vi "xcorr bkp.vi"(4 "shift":u8, 6 "N":u8, 7 "y":u32, 8 "x":u32, 9 "enable":bool, 10 "lag":u16) -> (1 "Rxy valid":bool, 2 "Rxy":u64, 3 "trigger":bool)   [LabVIEW 2017]
uses:
  <vilib>/rvi/FXPMathLib/basic elements/FxpDiscreteDelay/XNode/nifxpmath_DiscreteDelay.xnode
panel:
  in  "Pulse Energy":fxp<+,48,0>=0.99609375
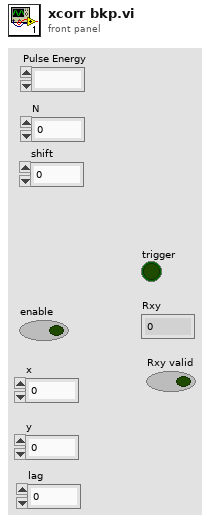
[diagram p1: front panel]
types:
  T1 = cluster{"Q":bool, "Q":bool, "Q":bool, "Q":bool, "Q":bool, "Q":bool, "Q":bool, "Q":bool, "Q":bool, "Q":bool, "Q":bool, "Q":bool, "valid":bool}
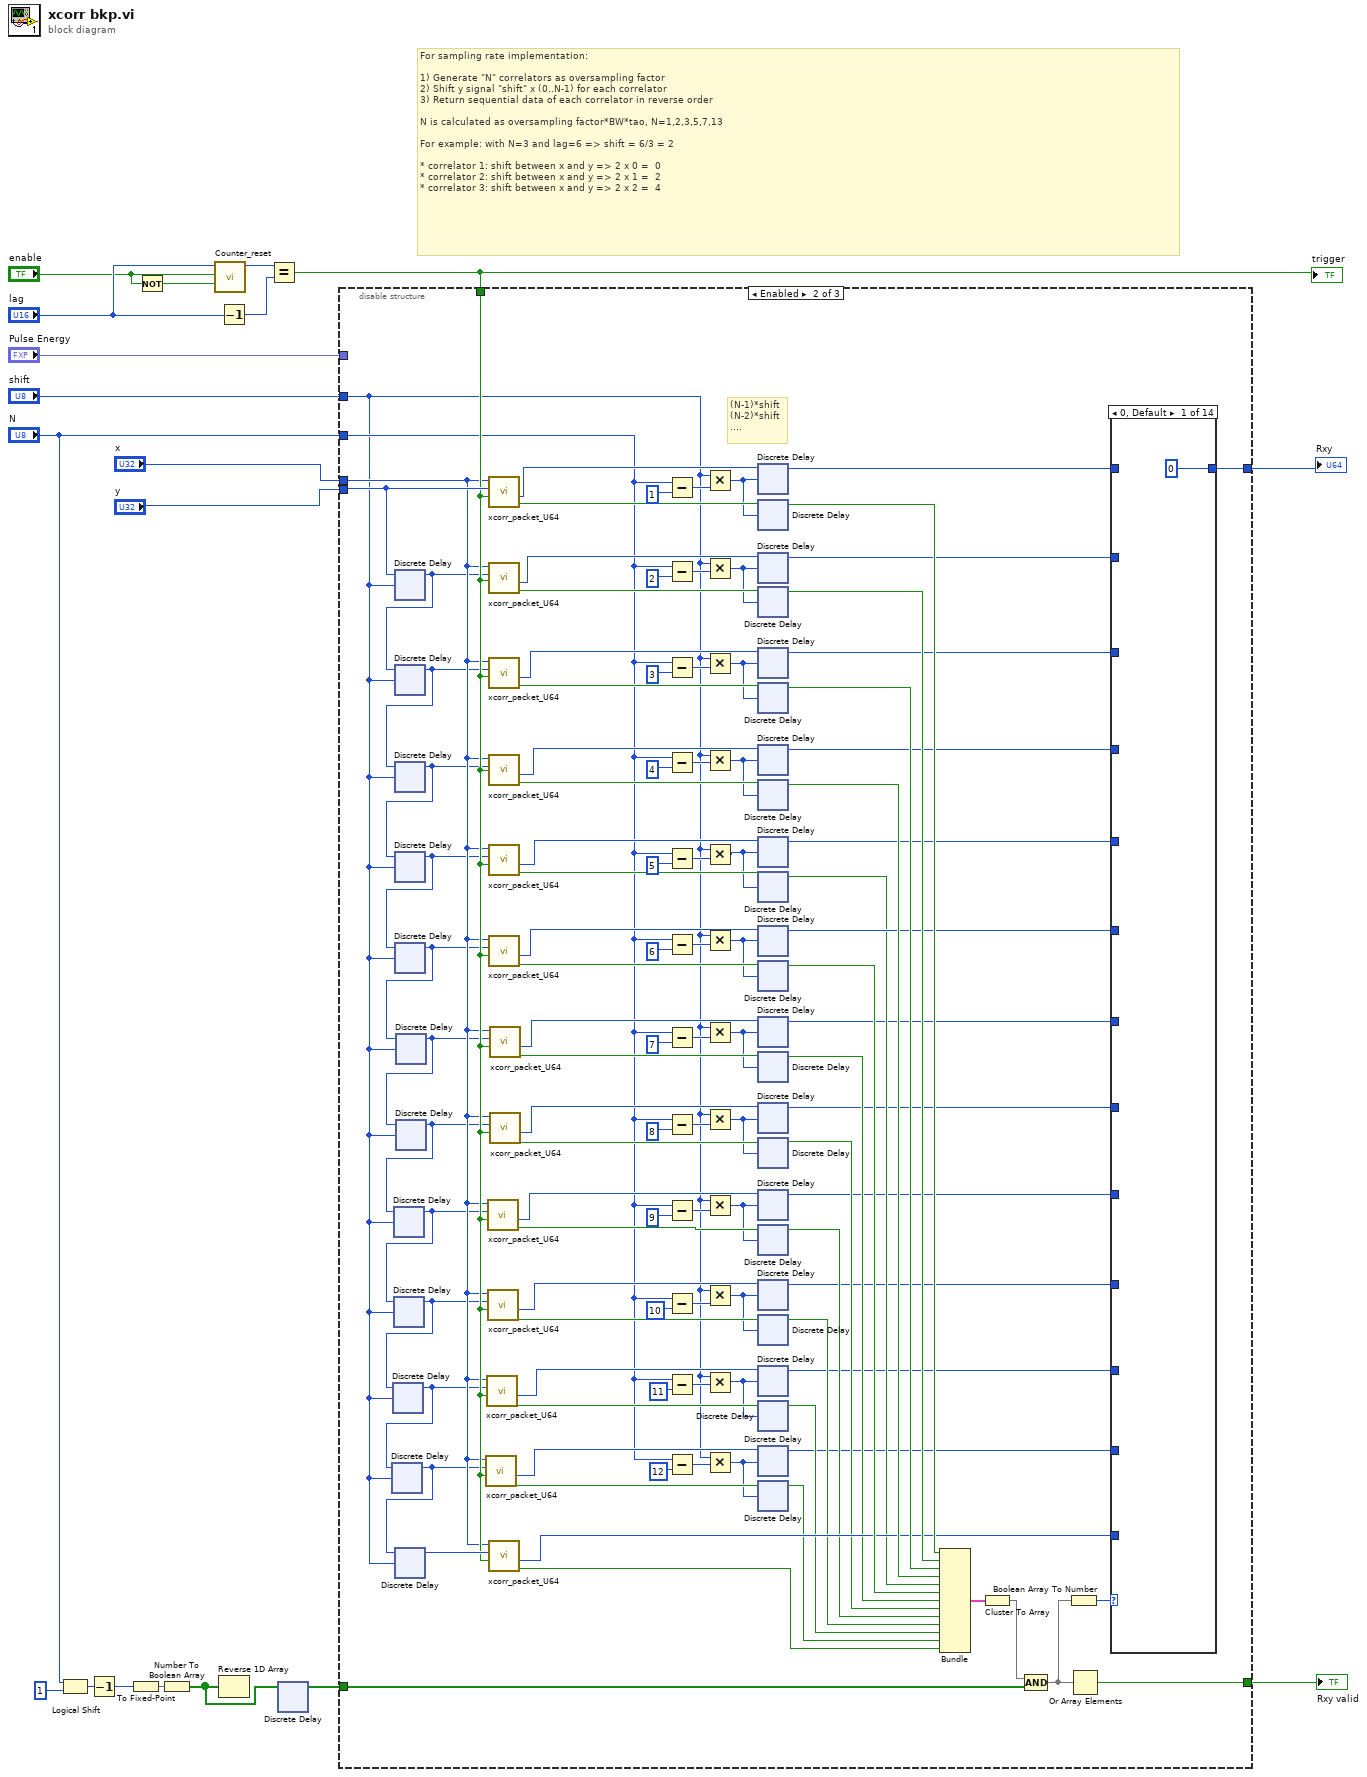
[diagram p0: block diagram]
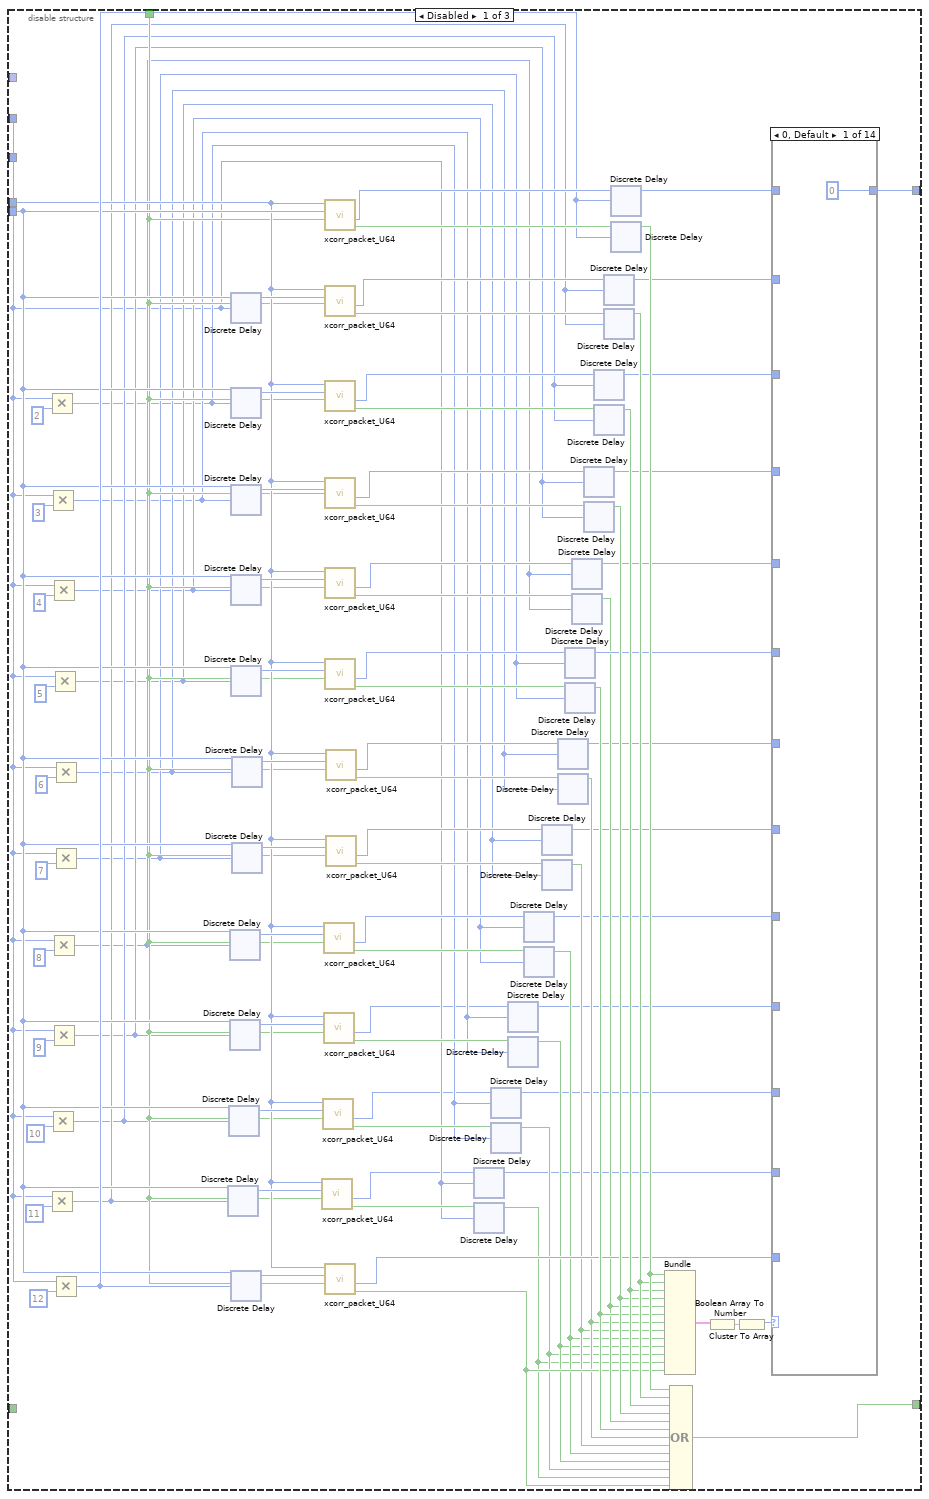
[diagram p2: hidden frame]
diagram:
  # "For sampling rate implementation:\n\n1) Generate \"N\" correlators as oversampling factor\n2) Shift y signal \"shift\" x (0..N-1) for each correlator\n3) Return sequential data of each correlator in reverse order\n\nN is calculated as oversampling factor*BW*tao, N=1,2,3,5,7,13\n\nFor example: with N=3 and lag=6 => shift = 6/3 = 2\n\n* correlator 1: shift between x and y => 2 x 0 =  0\n* correlator 2: shift between x and y => 2 x 1 =  2\n* correlator 3: shift between x and y => 2 x 2 =  4"
  n1 = Logical Shift(y="N", x=u16 1) -> (x << y=w7:u16)
  n2 = Decrement(x=w7) -> (x-1=w6:u16)
  n3 = To Fixed-Point(number=w6) -> (fixed-point=w5:fxp<+,13,13>)  [unwired: 1 in]
  n4 = Not(x="enable") -> (.not. x?=w17:bool)
  n5 = Number To Boolean Array(number=w5) -> (Boolean array=w2:bool[])
  n6 = call "Counter_reset.vi"("reset"=w17, "enable"="enable", "limit"="lag") -> ("count"=w18:u16)  [unwired: 8 in]
  n7 = Decrement(x="lag") -> (x-1=w15:u16)
  n8 = Reverse 1D Array(array=w2) -> ()  [unwired: 1 out]
  n9 = Equal?(x=w18, y=w15) -> (x = y?=w12:bool)
  "trigger" <- w12
  n10 = xnode ("Discrete Delay")("D"=w2) -> ("Q"=w9:bool[])
  n11 = disable-structure shown="Enabled" {
    disable-tunnel: [w112 w168 _] -> w19
    disable-tunnel: [w107 w233 _] -> w14
    disable-tunnel: "y" -> [w42 w191 _]
    disable-tunnel: "x" -> [w41 w180 _]
    disable-tunnel: w12 -> [w40 w190 _]
    disable-tunnel: "shift" -> [w28 w127 _]
    disable-tunnel: w9 -> [_ w167 _]
    disable-tunnel: "N" -> [_ w129 _]
    disable-tunnel: "Pulse Energy" -> [_ _ _]
    frame Disabled {
      n12 = Multiply(x=w28, y=u8 2 ("x")) -> (x*y=w29:u8)
      n13 = Multiply(x=w28, y=u8 11 ("x")) -> (x*y=w38:u8)
      n14 = Multiply(x=w28, y=u8 3 ("x")) -> (x*y=w30:u8)
      n15 = Multiply(x=w28, y=u8 10 ("x")) -> (x*y=w37:u8)
      n16 = Multiply(x=w28, y=u8 4 ("x")) -> (x*y=w31:u8)
      n17 = Multiply(x=w28, y=u8 8 ("x")) -> (x*y=w35:u8)
      n18 = Multiply(x=w28, y=u8 9 ("x")) -> (x*y=w36:u8)
      n19 = Multiply(x=w28, y=u8 5 ("x")) -> (x*y=w32:u8)
      n20 = Multiply(x=w28, y=u8 6 ("x")) -> (x*y=w33:u8)
      n21 = Multiply(x=w28, y=u8 7 ("x")) -> (x*y=w34:u8)
      n22 = Multiply(x=w28, y=u8 12 ("x")) -> (x*y=w78:u8)
      n23 = xnode ("Discrete Delay")("D"=w42, "n-1[0..255]"=w38) -> ("Q"=w44:u32)
      n24 = xnode ("Discrete Delay")("D"=w42, "n-1[0..255]"=w37) -> ("Q"=w51:u32)
      n25 = xnode ("Discrete Delay")("D"=w42, "n-1[0..255]"=w35) -> ("Q"=w57:u32)
      n26 = xnode ("Discrete Delay")("D"=w42, "n-1[0..255]"=w36) -> ("Q"=w54:u32)
      n27 = xnode ("Discrete Delay")("D"=w42, "n-1[0..255]"=w28) -> ("Q"=w111:u32)
      n28 = xnode ("Discrete Delay")("D"=w42, "n-1[0..255]"=w29) -> ("Q"=w105:u32)
      n29 = xnode ("Discrete Delay")("D"=w42, "n-1[0..255]"=w30) -> ("Q"=w103:u32)
      n30 = xnode ("Discrete Delay")("D"=w42, "n-1[0..255]"=w31) -> ("Q"=w101:u32)
      n31 = xnode ("Discrete Delay")("D"=w42, "n-1[0..255]"=w32) -> ("Q"=w87:u32)
      n32 = xnode ("Discrete Delay")("D"=w42, "n-1[0..255]"=w78) -> ("Q"=w79:u32)
      n33 = xnode ("Discrete Delay")("D"=w42, "n-1[0..255]"=w33) -> ("Q"=w72:u32)
      n34 = xnode ("Discrete Delay")("D"=w42, "n-1[0..255]"=w34) -> ("Q"=w62:u32)
      n35 = call "xcorr_packet_U64.vi"("x"=w41, "y"=w44, "trigger"=w40) -> ("out"=w20:u64, "valid"=w43:bool)  [unwired: 5 in]
      n36 = call "xcorr_packet_U64.vi"("x"=w41, "y"=w51, "trigger"=w40) -> ("out"=w21:u64, "valid"=w52:bool)  [unwired: 5 in]
      n37 = call "xcorr_packet_U64.vi"("x"=w41, "y"=w57, "trigger"=w40) -> ("out"=w59:u64, "valid"=w58:bool)  [unwired: 5 in]
      n38 = call "xcorr_packet_U64.vi"("x"=w41, "y"=w54, "trigger"=w40) -> ("out"=w22:u64, "valid"=w53:bool)  [unwired: 5 in]
      n39 = call "xcorr_packet_U64.vi"("x"=w41, "y"=w42, "trigger"=w40) -> ("out"=w110:u64, "valid"=w109:bool)  [unwired: 5 in]
      n40 = call "xcorr_packet_U64.vi"("x"=w41, "y"=w111, "trigger"=w40) -> ("out"=w93:u64, "valid"=w98:bool)  [unwired: 5 in]
      n41 = call "xcorr_packet_U64.vi"("x"=w41, "y"=w105, "trigger"=w40) -> ("out"=w92:u64, "valid"=w97:bool)  [unwired: 5 in]
      n42 = call "xcorr_packet_U64.vi"("x"=w41, "y"=w103, "trigger"=w40) -> ("out"=w90:u64, "valid"=w95:bool)  [unwired: 5 in]
      n43 = call "xcorr_packet_U64.vi"("x"=w41, "y"=w101, "trigger"=w40) -> ("out"=w82:u64, "valid"=w76:bool)  [unwired: 5 in]
      n44 = call "xcorr_packet_U64.vi"("x"=w41, "y"=w87, "trigger"=w40) -> ("out"=w84:u64, "valid"=w86:bool)  [unwired: 5 in]
      n45 = call "xcorr_packet_U64.vi"("x"=w41, "y"=w79, "trigger"=w40) -> ("out"=w77:u64, "valid"=w69:bool)  [unwired: 5 in]
      n46 = call "xcorr_packet_U64.vi"("x"=w41, "y"=w72, "trigger"=w40) -> ("out"=w74:u64, "valid"=w73:bool)  [unwired: 5 in]
      n47 = call "xcorr_packet_U64.vi"("x"=w41, "y"=w62, "trigger"=w40) -> ("out"=w60:u64, "valid"=w61:bool)  [unwired: 5 in]
      n48 = xnode ("Discrete Delay")("D"=w20, "n-1[0..255]"=w28) -> ("Q"=w24:u64)
      n49 = xnode ("Discrete Delay")("D"=w43, "n-1[0..255]"=w28) -> ("Q"=w39:bool)
      n50 = xnode ("Discrete Delay")("D"=w21, "n-1[0..255]"=w29) -> ("Q"=w25:u64)
      n51 = xnode ("Discrete Delay")("D"=w52, "n-1[0..255]"=w29) -> ("Q"=w46:bool)
      n52 = xnode ("Discrete Delay")("D"=w22, "n-1[0..255]"=w30) -> ("Q"=w26:u64)
      n53 = xnode ("Discrete Delay")("D"=w53, "n-1[0..255]"=w30) -> ("Q"=w47:bool)
      n54 = xnode ("Discrete Delay")("D"=w59, "n-1[0..255]"=w31) -> ("Q"=w27:u64)
      n55 = xnode ("Discrete Delay")("D"=w58, "n-1[0..255]"=w31) -> ("Q"=w48:bool)
      n56 = xnode ("Discrete Delay")("D"=w60, "n-1[0..255]"=w32) -> ("Q"=w23:u64)
      n57 = xnode ("Discrete Delay")("D"=w61, "n-1[0..255]"=w32) -> ("Q"=w49:bool)
      n58 = xnode ("Discrete Delay")("D"=w74, "n-1[0..255]"=w33) -> ("Q"=w70:u64)
      n59 = xnode ("Discrete Delay")("D"=w73, "n-1[0..255]"=w33) -> ("Q"=w67:bool)
      n60 = xnode ("Discrete Delay")("D"=w84, "n-1[0..255]"=w34) -> ("Q"=w83:u64)
      n61 = xnode ("Discrete Delay")("D"=w86, "n-1[0..255]"=w34) -> ("Q"=w85:bool)
      n62 = xnode ("Discrete Delay")("D"=w82, "n-1[0..255]"=w35) -> ("Q"=w81:u64)
      n63 = xnode ("Discrete Delay")("D"=w76, "n-1[0..255]"=w35) -> ("Q"=w75:bool)
      n64 = xnode ("Discrete Delay")("D"=w90, "n-1[0..255]"=w36) -> ("Q"=w89:u64)
      n65 = xnode ("Discrete Delay")("D"=w95, "n-1[0..255]"=w36) -> ("Q"=w94:bool)
      n66 = xnode ("Discrete Delay")("D"=w92, "n-1[0..255]"=w37) -> ("Q"=w91:u64)
      n67 = xnode ("Discrete Delay")("D"=w97, "n-1[0..255]"=w37) -> ("Q"=w96:bool)
      n68 = xnode ("Discrete Delay")("D"=w93, "n-1[0..255]"=w38) -> ("Q"=w68:u64)
      n69 = xnode ("Discrete Delay")("D"=w98, "n-1[0..255]"=w38) -> ("Q"=w99:bool)
      n70 = xnode ("Discrete Delay")("D"=w110, "n-1[0..255]"=w78) -> ("Q"=w108:u64)
      n71 = xnode ("Discrete Delay")("D"=w109, "n-1[0..255]"=w78) -> ("Q"=w100:bool)
      n72 = Bundle("Q"=w100, "Q"=w99, "Q"=w96, "Q"=w94, "Q"=w75, "Q"=w85, "Q"=w67, "Q"=w49, "Q"=w48, "Q"=w47, "Q"=w46, "Q"=w39, "valid"=w69) -> (w66:T1)  [unwired: 1 in]
      n73 = Compound Arithmetic op=OR(w100, w99, w96, w94, w75, w85, w67, w49, w48, w47, w46, w39, w69) -> (w112:bool)
      n74 = Cluster To Array(cluster=w66) -> (array=w64:bool[])
      n75 = Boolean Array To Number(Boolean array=w64) -> (number=w65:u16)
      n76 = case shown="0, Default" w65 {
        tunnel: [u64 0 ("out") w114 w115 w116 w117 w118 w119 w120 w121 w122 w123 w124 w125 w126] -> w107
        tunnel: w108 -> [_ w114 _ _ _ _ _ _ _ _ _ _ _ _]
        tunnel: w68 -> [_ _ w115 _ _ _ _ _ _ _ _ _ _ _]
        tunnel: w91 -> [_ _ _ w116 _ _ _ _ _ _ _ _ _ _]
        tunnel: w89 -> [_ _ _ _ w117 _ _ _ _ _ _ _ _ _]
        tunnel: w81 -> [_ _ _ _ _ w118 _ _ _ _ _ _ _ _]
        tunnel: w83 -> [_ _ _ _ _ _ w119 _ _ _ _ _ _ _]
        tunnel: w77 -> [_ _ _ _ _ _ _ _ _ _ _ _ _ w126]
        tunnel: w70 -> [_ _ _ _ _ _ _ w120 _ _ _ _ _ _]
        tunnel: w23 -> [_ _ _ _ _ _ _ _ w121 _ _ _ _ _]
        tunnel: w27 -> [_ _ _ _ _ _ _ _ _ w122 _ _ _ _]
        tunnel: w26 -> [_ _ _ _ _ _ _ _ _ _ w123 _ _ _]
        tunnel: w25 -> [_ _ _ _ _ _ _ _ _ _ _ w124 _ _]
        tunnel: w24 -> [_ _ _ _ _ _ _ _ _ _ _ _ w125 _]
        frame 0, Default {
        }
        frame 1 {
        }
        frame 2 {
        }
        frame 4 {
        }
        frame 8 {
        }
        frame 16 {
        }
        frame 32 {
        }
        frame 64 {
        }
        frame 128 {
        }
        frame 256 {
        }
        frame 512 {
        }
        frame 1024 {
        }
        frame 2048 {
        }
        frame 4096 {
        }
      }
    }
    frame Enabled {
      # "(N-1)*shift\n(N-2)*shift\n...."
      n77 = xnode ("Discrete Delay")("D"=w191, "n-1[0..255]"=w127) -> ("Q"=w169:u32)
      n78 = xnode ("Discrete Delay")("D"=w169, "n-1[0..255]"=w127) -> ("Q"=w179:u32)
      n79 = xnode ("Discrete Delay")("D"=w179, "n-1[0..255]"=w127) -> ("Q"=w178:u32)
      n80 = xnode ("Discrete Delay")("D"=w178, "n-1[0..255]"=w127) -> ("Q"=w177:u32)
      n81 = xnode ("Discrete Delay")("D"=w177, "n-1[0..255]"=w127) -> ("Q"=w176:u32)
      n82 = xnode ("Discrete Delay")("D"=w176, "n-1[0..255]"=w127) -> ("Q"=w175:u32)
      n83 = xnode ("Discrete Delay")("D"=w175, "n-1[0..255]"=w127) -> ("Q"=w174:u32)
      n84 = xnode ("Discrete Delay")("D"=w174, "n-1[0..255]"=w127) -> ("Q"=w173:u32)
      n85 = xnode ("Discrete Delay")("D"=w173, "n-1[0..255]"=w127) -> ("Q"=w172:u32)
      n86 = xnode ("Discrete Delay")("D"=w172, "n-1[0..255]"=w127) -> ("Q"=w171:u32)
      n87 = xnode ("Discrete Delay")("D"=w171, "n-1[0..255]"=w127) -> ("Q"=w170:u32)
      n88 = xnode ("Discrete Delay")("D"=w170, "n-1[0..255]"=w127) -> ("Q"=w214:u32)
      n89 = call "xcorr_packet_U64.vi"("x"=w180, "y"=w170, "trigger"=w190) -> ("out"=w181:u64, "valid"=w192:bool)  [unwired: 5 in]
      n90 = call "xcorr_packet_U64.vi"("x"=w180, "y"=w171, "trigger"=w190) -> ("out"=w182:u64, "valid"=w197:bool)  [unwired: 5 in]
      n91 = call "xcorr_packet_U64.vi"("x"=w180, "y"=w173, "trigger"=w190) -> ("out"=w200:u64, "valid"=w199:bool)  [unwired: 5 in]
      n92 = call "xcorr_packet_U64.vi"("x"=w180, "y"=w172, "trigger"=w190) -> ("out"=w183:u64, "valid"=w198:bool)  [unwired: 5 in]
      n93 = call "xcorr_packet_U64.vi"("x"=w180, "y"=w191, "trigger"=w190) -> ("out"=w236:u64, "valid"=w235:bool)  [unwired: 5 in]
      n94 = call "xcorr_packet_U64.vi"("x"=w180, "y"=w169, "trigger"=w190) -> ("out"=w225:u64, "valid"=w230:bool)  [unwired: 5 in]
      n95 = call "xcorr_packet_U64.vi"("x"=w180, "y"=w179, "trigger"=w190) -> ("out"=w224:u64, "valid"=w229:bool)  [unwired: 5 in]
      n96 = call "xcorr_packet_U64.vi"("x"=w180, "y"=w178, "trigger"=w190) -> ("out"=w222:u64, "valid"=w227:bool)  [unwired: 5 in]
      n97 = call "xcorr_packet_U64.vi"("x"=w180, "y"=w177, "trigger"=w190) -> ("out"=w216:u64, "valid"=w212:bool)  [unwired: 5 in]
      n98 = call "xcorr_packet_U64.vi"("x"=w180, "y"=w176, "trigger"=w190) -> ("out"=w218:u64, "valid"=w220:bool)  [unwired: 5 in]
      n99 = call "xcorr_packet_U64.vi"("x"=w180, "y"=w214, "trigger"=w190) -> ("out"=w213:u64, "valid"=w207:bool)  [unwired: 5 in]
      n100 = call "xcorr_packet_U64.vi"("x"=w180, "y"=w175, "trigger"=w190) -> ("out"=w210:u64, "valid"=w209:bool)  [unwired: 5 in]
      n101 = call "xcorr_packet_U64.vi"("x"=w180, "y"=w174, "trigger"=w190) -> ("out"=w201:u64, "valid"=w202:bool)  [unwired: 5 in]
      n102 = Subtract(x=w129, y=u8 1 ("x")) -> (x-y=w163:u8)
      n103 = Subtract(x=w129, y=u8 2 ("x")) -> (x-y=w161:u8)
      n104 = Subtract(x=w129, y=u8 3 ("x")) -> (x-y=w159:u8)
      n105 = Subtract(x=w129, y=u8 4 ("x")) -> (x-y=w157:u8)
      n106 = Subtract(x=w129, y=u8 5 ("x")) -> (x-y=w155:u8)
      n107 = Subtract(x=w129, y=u8 6 ("x")) -> (x-y=w153:u8)
      n108 = Subtract(x=w129, y=u8 7 ("x")) -> (x-y=w151:u8)
      n109 = Subtract(x=w129, y=u8 8 ("x")) -> (x-y=w149:u8)
      n110 = Subtract(x=w129, y=u8 9 ("x")) -> (x-y=w147:u8)
      n111 = Subtract(x=w129, y=u8 10 ("x")) -> (x-y=w145:u8)
      n112 = Subtract(x=w129, y=u8 11 ("x")) -> (x-y=w143:u8)
      n113 = Subtract(x=w129, y=u8 12 ("x")) -> (x-y=w131:u8)
      n114 = Multiply(x=w127, y=w163) -> (x*y=w142:u8)
      n115 = Multiply(x=w127, y=w161) -> (x*y=w141:u8)
      n116 = Multiply(x=w127, y=w159) -> (x*y=w140:u8)
      n117 = Multiply(x=w127, y=w157) -> (x*y=w139:u8)
      n118 = Multiply(x=w127, y=w155) -> (x*y=w138:u8)
      n119 = Multiply(x=w127, y=w153) -> (x*y=w137:u8)
      n120 = Multiply(x=w127, y=w151) -> (x*y=w136:u8)
      n121 = Multiply(x=w127, y=w149) -> (x*y=w135:u8)
      n122 = Multiply(x=w127, y=w147) -> (x*y=w134:u8)
      n123 = Multiply(x=w127, y=w145) -> (x*y=w133:u8)
      n124 = Multiply(x=w127, y=w143) -> (x*y=w132:u8)
      n125 = Multiply(x=w127, y=w131) -> (x*y=w128:u8)
      n126 = xnode ("Discrete Delay")("D"=w236, "n-1[0..255]"=w142) -> ("Q"=w234:u64)
      n127 = xnode ("Discrete Delay")("D"=w235, "n-1[0..255]"=w142) -> ("Q"=w232:bool)
      n128 = xnode ("Discrete Delay")("D"=w225, "n-1[0..255]"=w141) -> ("Q"=w206:u64)
      n129 = xnode ("Discrete Delay")("D"=w230, "n-1[0..255]"=w141) -> ("Q"=w231:bool)
      n130 = xnode ("Discrete Delay")("D"=w224, "n-1[0..255]"=w140) -> ("Q"=w223:u64)
      n131 = xnode ("Discrete Delay")("D"=w229, "n-1[0..255]"=w140) -> ("Q"=w228:bool)
      n132 = xnode ("Discrete Delay")("D"=w222, "n-1[0..255]"=w139) -> ("Q"=w221:u64)
      n133 = xnode ("Discrete Delay")("D"=w227, "n-1[0..255]"=w139) -> ("Q"=w226:bool)
      n134 = xnode ("Discrete Delay")("D"=w216, "n-1[0..255]"=w138) -> ("Q"=w215:u64)
      n135 = xnode ("Discrete Delay")("D"=w212, "n-1[0..255]"=w138) -> ("Q"=w211:bool)
      n136 = xnode ("Discrete Delay")("D"=w218, "n-1[0..255]"=w137) -> ("Q"=w217:u64)
      n137 = xnode ("Discrete Delay")("D"=w220, "n-1[0..255]"=w137) -> ("Q"=w219:bool)
      n138 = xnode ("Discrete Delay")("D"=w210, "n-1[0..255]"=w136) -> ("Q"=w208:u64)
      n139 = xnode ("Discrete Delay")("D"=w209, "n-1[0..255]"=w136) -> ("Q"=w205:bool)
      n140 = xnode ("Discrete Delay")("D"=w201, "n-1[0..255]"=w135) -> ("Q"=w184:u64)
      n141 = xnode ("Discrete Delay")("D"=w202, "n-1[0..255]"=w135) -> ("Q"=w196:bool)
      n142 = xnode ("Discrete Delay")("D"=w200, "n-1[0..255]"=w134) -> ("Q"=w188:u64)
      n143 = xnode ("Discrete Delay")("D"=w199, "n-1[0..255]"=w134) -> ("Q"=w195:bool)
      n144 = xnode ("Discrete Delay")("D"=w183, "n-1[0..255]"=w133) -> ("Q"=w187:u64)
      n145 = xnode ("Discrete Delay")("D"=w198, "n-1[0..255]"=w133) -> ("Q"=w194:bool)
      n146 = xnode ("Discrete Delay")("D"=w182, "n-1[0..255]"=w132) -> ("Q"=w186:u64)
      n147 = xnode ("Discrete Delay")("D"=w197, "n-1[0..255]"=w132) -> ("Q"=w193:bool)
      n148 = xnode ("Discrete Delay")("D"=w181, "n-1[0..255]"=w128) -> ("Q"=w185:u64)
      n149 = xnode ("Discrete Delay")("D"=w192, "n-1[0..255]"=w128) -> ("Q"=w189:bool)
      n150 = Bundle("Q"=w232, "Q"=w231, "Q"=w228, "Q"=w226, "Q"=w211, "Q"=w219, "Q"=w205, "Q"=w196, "Q"=w195, "Q"=w194, "Q"=w193, "Q"=w189, "valid"=w207) -> (w204:T1)  [unwired: 1 in]
      n151 = Cluster To Array(cluster=w204) -> (array=w166:bool[])
      n152 = Compound Arithmetic op=AND(w166, w167) -> (w165:bool[])
      n153 = Boolean Array To Number(Boolean array=w165) -> (number=w203:u16)
      n154 = Or Array Elements(Boolean array=w165) -> (logical OR=w168:bool)
      n155 = case shown="0, Default" w203 {
        tunnel: [u64 0 ("out") w238 w239 w240 w241 w242 w243 w244 w245 w246 w247 w248 w249 w250] -> w233
        tunnel: w234 -> [_ w238 _ _ _ _ _ _ _ _ _ _ _ _]
        tunnel: w206 -> [_ _ w239 _ _ _ _ _ _ _ _ _ _ _]
        tunnel: w223 -> [_ _ _ w240 _ _ _ _ _ _ _ _ _ _]
        tunnel: w221 -> [_ _ _ _ w241 _ _ _ _ _ _ _ _ _]
        tunnel: w215 -> [_ _ _ _ _ w242 _ _ _ _ _ _ _ _]
        tunnel: w217 -> [_ _ _ _ _ _ w243 _ _ _ _ _ _ _]
        tunnel: w213 -> [_ _ _ _ _ _ _ _ _ _ _ _ _ w250]
        tunnel: w208 -> [_ _ _ _ _ _ _ w244 _ _ _ _ _ _]
        tunnel: w184 -> [_ _ _ _ _ _ _ _ w245 _ _ _ _ _]
        tunnel: w188 -> [_ _ _ _ _ _ _ _ _ w246 _ _ _ _]
        tunnel: w187 -> [_ _ _ _ _ _ _ _ _ _ w247 _ _ _]
        tunnel: w186 -> [_ _ _ _ _ _ _ _ _ _ _ w248 _ _]
        tunnel: w185 -> [_ _ _ _ _ _ _ _ _ _ _ _ w249 _]
        frame 0, Default {
        }
        frame 1 {
        }
        frame 2 {
        }
        frame 4 {
        }
        frame 8 {
        }
        frame 16 {
        }
        frame 32 {
        }
        frame 64 {
        }
        frame 128 {
        }
        frame 256 {
        }
        frame 512 {
        }
        frame 1024 {
        }
        frame 2048 {
        }
        frame 4096 {
        }
      }
    }
    frame Disabled {
    }
  }
  "Rxy valid" <- w19
  "Rxy" <- w14
